vi "Save.vi"(8 "error in":errorcluster, 11 "state in":T1) -> (0 "error out":errorcluster, 3 "state out":T1)   [LabVIEW 2013, in "RT Temperature Controller.lvlib"]
uses:
  RT Temperature Controller.lvlib
  Controls/StateCluster.ctl
  <vilib>/NI/Tag Bus Data Framework/Configuration Editor/Classes/SystemConfigRepo/SystemConfigRepo.lvclass
  <vilib>/CEF_TreeControl/Node/NodeRef.ctl
  <vilib>/CEF_TreeControl/Node/NISE_CEF_Node.lvclass
  <vilib>/CEF_TreeControl/Node/UserEventRef.ctl
  <vilib>/CEF_TreeControl/Controls/EventCluster.ctl
  SplashScreen/splash screen.ctl
  SplashScreen/notifier data.ctl
  <vilib>/CEF_TreeControl/NISE_CEF_TreeControl.lvlib
  SplashScreen/splash screen.lvlib
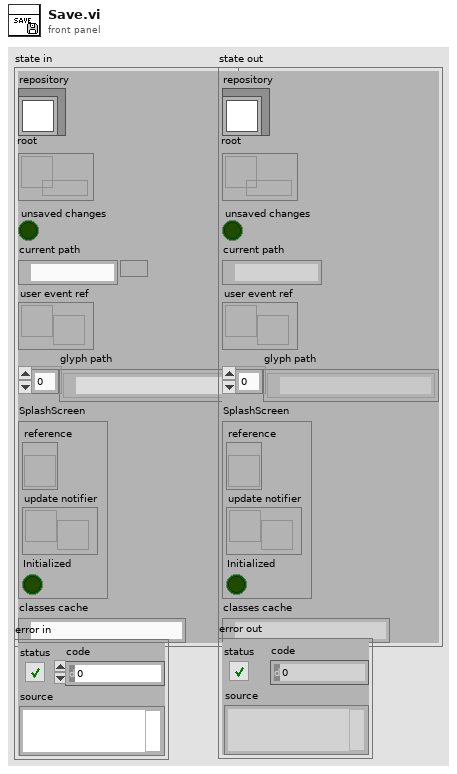
[diagram p1: front panel]
types:
  T1 = typedef "RT Temperature Controller.lvlib/StateCluster.ctl" = cluster{"repository":refnum<class "SystemConfigRepo.lvclass">, "root":T2, "unsaved changes":bool, "current path":path, "user event ref":T3, "glyph path":path[], "SplashScreen":T4, "classes cache":path}
  T2 = typedef "NISE_CEF_Node.lvclass/NodeRef.ctl" = refnum<data-value>
  T3 = typedef "NISE_CEF_Node.lvclass/UserEventRef.ctl" = refnum<user-event>
  T4 = typedef "RT Temperature Controller.lvlib/splash screen.lvlib/splash screen.ctl" = cluster{"reference":refnum<vi>, "update notifier":refnum<notifier>, "Initialized":bool}
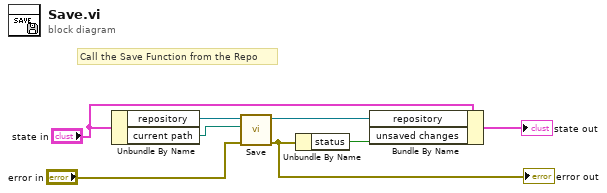
[diagram p0: block diagram]
diagram:
  # "Call the Save Function from the Repo"
  n1 = Unbundle By Name("state in") -> ("repository"=w8:refnum<class "SystemConfigRepo.lvclass">, "current path"=w2:path)
  n2 = call-dynamic "Save.vi"("error in"="error in", "file path"=w2, "SystemConfigRepo in"=w8) -> ("error out"=w4:errorcluster, "SystemConfigRepo out"=w1:refnum<class "SystemConfigRepo.lvclass">)  [unwired: 7 in]
  "error out" <- w4
  n3 = Unbundle By Name(w4) -> ("status"=w3:bool)
  n4 = Bundle By Name(cluster="state in", "repository"=w1, "unsaved changes"=w3) -> (→"state out":T1)
